vi "Get Handler Event.vi"(8 "error in":errorcluster, 11 "Name":string) -> (0 "error out":errorcluster, 3 "Logging Event":refnum<user-event>)   [LabVIEW 2020, in "hse-logger.lvlib"]
doc: "Returns the User Event from the Handler specified by name. The name must correspond to a ``UserEventHandler``.\nIf name was not found, returns a basis handler without functionality and raise an error \"510802 - Handler name not found\".\n\n____\nHAMPEL SOFTWARE ENGINEERING v2.0.6 (2021-04-15 11:38)"
uses:
  hse-logger.lvlib
  Handler/UserEventHandler/UserEventHandler.lvclass
  LogRecord/LogRecord.lvclass
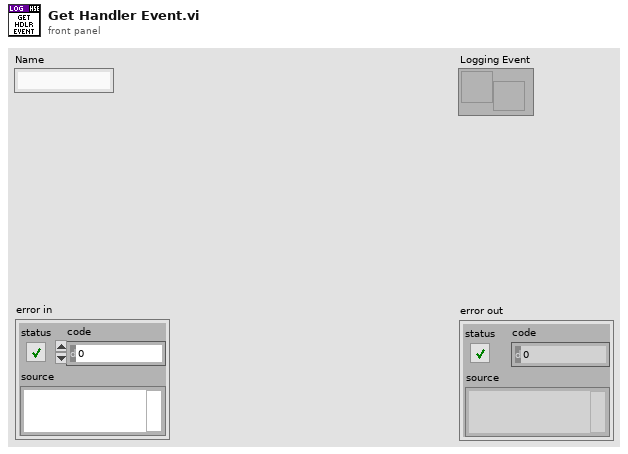
[diagram p1: front panel]
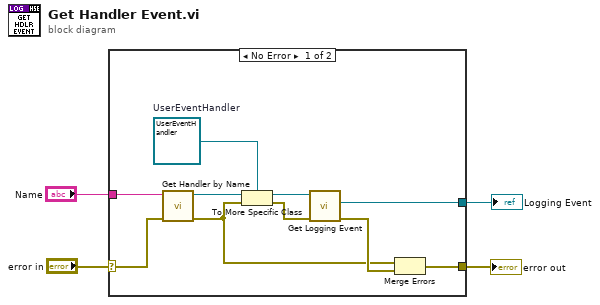
[diagram p0: block diagram]
diagram:
  n1 = case shown="No Error" "error in" {
    selector: "error in" -> [w14 w15]
    tunnel: [w6 w15] -> w3
    tunnel: "Name" -> [w13 _]
    tunnel: [w8 _] -> w1
    frame No Error {
      w9 = refnum<class "UserEventHandler.lvclass"> refnum  # UserEventHandler
      n2 = call "Get Handler by Name.vi"("error in"=w14, "Name"=w13) -> ("error out"=w5:errorcluster, "Handler out"=w10:refnum<class "Handler.lvclass">)  [unwired: 8 in]
      n3 = To More Specific Class(target class=w9, reference=w10, error in=w5) -> (specific class reference=w12:refnum<class "UserEventHandler.lvclass">, error out=w11:errorcluster)
      n4 = call-dynamic "Get Logging Event.vi"("error in"=w11, "UserEventHandler in"=w12) -> ("error out"=w7:errorcluster, "Logging Event"=w8:refnum<user-event>)  [unwired: 7 in, 1 out]
      n5 = Merge Errors(w5, w7) -> (w6:errorcluster)
    }
    frame Error {
    }
  }
  "error out" <- w3
  "Logging Event" <- w1
